vi "tcpExampleServer.vi"() -> ()   [LabVIEW 2014]
uses:
  typedefs/clientStatus.ctl
  typedefs/clientConfiguration.ctl
panel:
  out "server status":T1
  out "receive client->server":string
  in  "transmit server->client":string
  in  "stop":bool
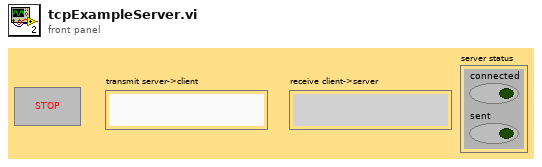
[diagram p1: front panel]
types:
  T1 = typedef "clientStatus.ctl" = cluster{"connected":bool, "sent":bool}
  T2 = typedef "clientConfiguration.ctl" = cluster{"client ID":string, "remote host":string, "local port":u16, "remote port":u16}
  T3 = cluster{"status":cluster{"queue":refnum<queue>, "error out":errorcluster}, "receive":cluster{"queue":refnum<queue>, "error out":errorcluster}, "transmit":cluster{"queue":refnum<queue>, "error out":errorcluster}, "shutdown":cluster{"queue":refnum<queue>, "error out":errorcluster}}
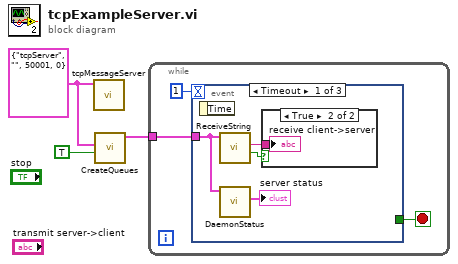
[diagram p0: block diagram]
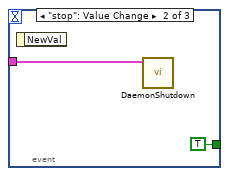
[diagram p3: hidden frame]
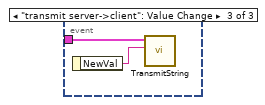
[diagram p4: hidden frame]
diagram:
  w3 = T2 {"client ID"="tcpServer", "remote host"="", "local port"=50001, "remote port"=0} ("client configuration")
  n1 = call "tcpMessageServer.vi"("server configuration"=w3) -> ()  [unwired: 10 in, 1 out]
  n2 = call "CreateQueues.vi"("create if not found? (T)"=TRUE, "client configuration"=w3) -> ("output cluster"=w1:T3)  [unwired: 9 in]
  n3 = while {
    tunnel: w1 -> [w5]
    stop <- w6 stop-if-true
    n4 = event shown="[0] Timeout" {
      selector: _ -> [_ _ _]
      dyn-events: _ -> [_ _ _]
      timeout: 1 -> [_ _ _]
      tunnel: [_ TRUE _] -> w6
      tunnel: w5 -> [w9 w12 w15]
      event Timeout {
        n5 = event-data() -> ()  [unwired: 1 in, 1 out]
        n6 = call "ReceiveString.vi"("queue cluster"=w9) -> ("new value"=w7:bool, "received string"=w10:string)  [unwired: 7 in, 2 out]
        n7 = call "DaemonStatus.vi"("queue cluster"=w9) -> ("status"=→"server status":T1)  [unwired: 8 in, 2 out]
        n8 = case shown="True" w7 {
          tunnel: w10 -> [_ w11]
          frame False {
          }
          frame True {
            "receive client->server" <- w11
          }
        }
      }
      event "stop": Value Change {
        n9 = event-data() -> ()  [unwired: 1 in, 1 out]
        n10 = call "DaemonShutdown.vi"("queue cluster"=w12) -> ()  [unwired: 9 in, 2 out]
      }
      event "transmit server->client": Value Change {
        n11 = event-data() -> ("NewVal"=w14:string)  [unwired: 1 in]
        n12 = call "TransmitString.vi"("string to transmit"=w14, "queue cluster"=w15) -> ()  [unwired: 8 in, 2 out]
      }
    }
  }
